vi "roboRIO TCP Client.vi"() -> ()   [LabVIEW 2025]
doc: "The UDP protocol differs from TCP in that there is no error-checking with the packets of information that are sent, and thus no guarantee whatsoever that an intended recipient will actually receive a given piece of data.\n\nUDP does offer the ability to \"broadcast\" data across a network--simply specify an IP Address of all ones (255.255.255.255) to attempt to broadcast information network-wide. Keep in mind that routers and other network hardware will generally refuse to forward the broadcast beyond certain points, so the extent of the broadcast will in practice be limited."
uses:
  roboRIO TCP Main States.ctl
panel:
  in  "Log?":bool
  out "Message Log":string[](array[string])
  out "String length":i32
  out "data string":string
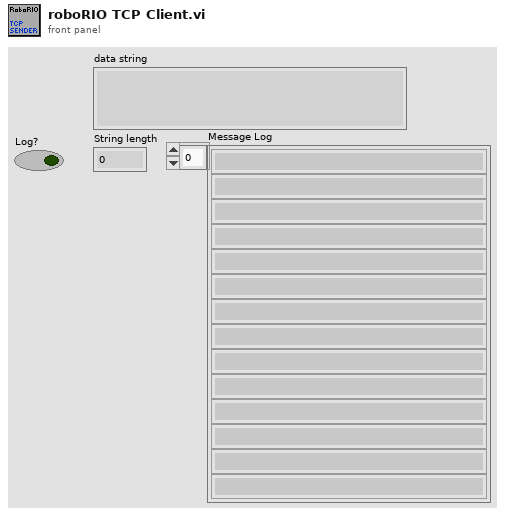
[diagram p1: front panel]
types:
  T1 = typedef "roboRIO TCP Main States.ctl" = enum16{"Message Dispatcher", "INI", "Read Data", "Send Data", "TCP Close", "TCP Open", "Exit"}
  T2 = typedef "Event Setup Types.ctl" = enum16{"Default", "Camera Loop Started", "GreyScale", "Reset Camera Settings", "Reset Team Number", "Save Data", "Setting Changed", "Update Video Mode", "Video Mode Changed", "Exit"}
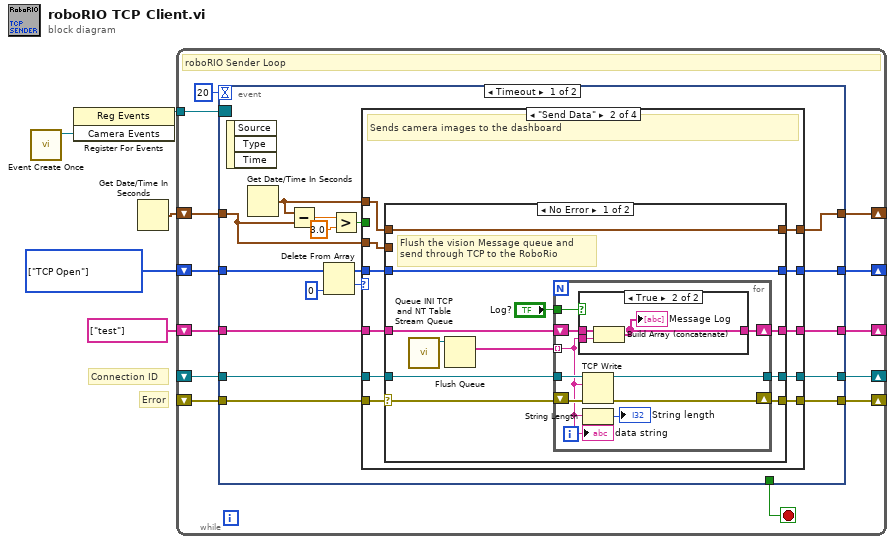
[diagram p0: block diagram]
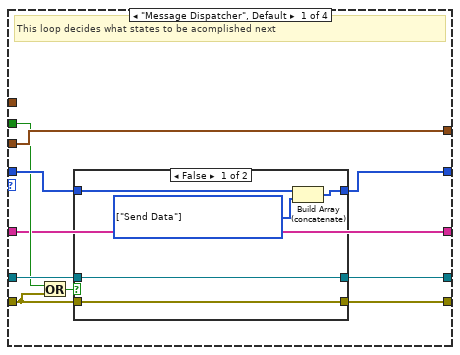
[diagram p2: hidden frame]
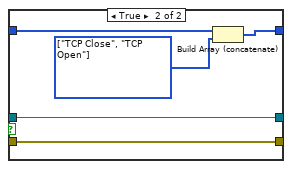
[diagram p3: hidden frame]
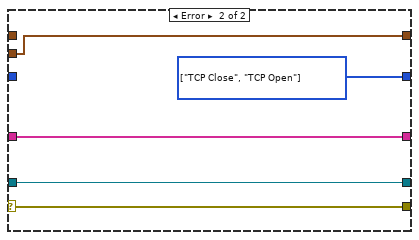
[diagram p5: hidden frame]
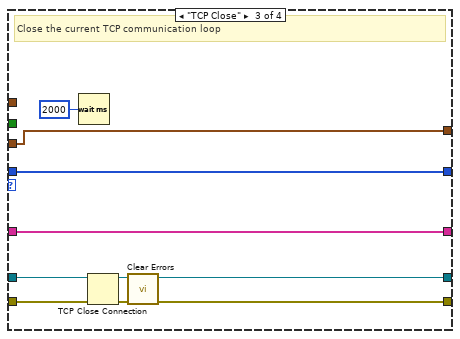
[diagram p6: hidden frame]
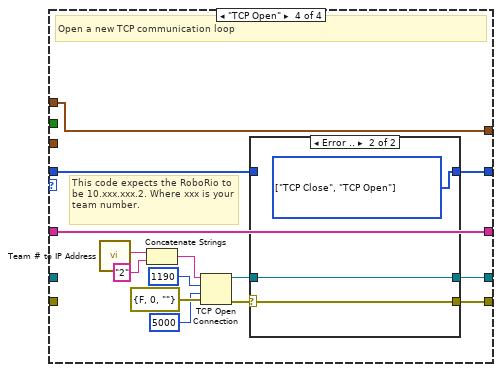
[diagram p7: hidden frame]
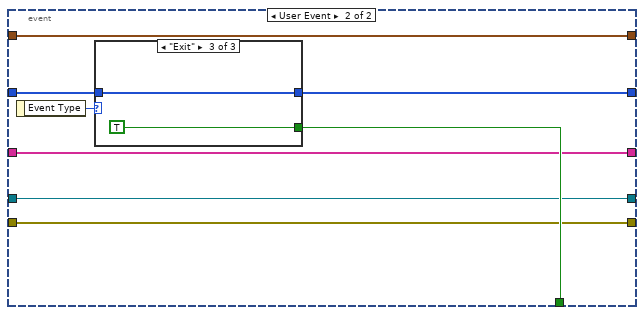
[diagram p9: hidden frame]
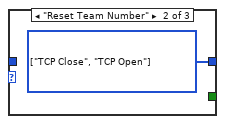
[diagram p11: hidden frame]
diagram:
  w5 = T1[] [enum."TCP Open"] items=["Message Dispatcher", "INI", "Read Data", "Send Data", "TCP Close", "TCP Open", "Exit"]
  # "Error"
  # "Connection ID"
  n1 = call "Event Create Once.vi"() -> ("Camera Events"=w3:refnum<user-event>)  [unwired: 10 in, 1 out]
  n2 = register-events(w3) -> (reference out=w2:refnum<event-registration>)  [unwired: 2 in, 1 out]
  n3 = Get Date/Time In Seconds() -> (seconds since 1Jan1904=w4:timestamp)
  n4 = while {
    shift-right: [w13] -> _
    shift-left: w5 -> [w14]
    shift-right: [w18] -> _
    shift-left: _ -> [w16]
    shift-right: [w17] -> _
    shift-left: _ -> [w15]
    shift-right: [w11] -> _
    shift-left: w4 -> [w10]
    tunnel: w2 -> [w9]
    shift-right: [w6] -> _
    shift-left: string[] ["test"] -> [w7]
    stop <- w12 stop-if-true
    # "roboRIO Sender Loop"
    n5 = event shown="[0] Timeout" {
      selector: w9 -> [_ _]
      dyn-events: _ -> [_ _]
      timeout: 20 -> [_ _]
      tunnel: [w35 w128] -> w18
      tunnel: [w34 w127] -> w17
      tunnel: w16 -> [w33 w128]
      tunnel: w15 -> [w20 w127]
      tunnel: w14 -> [w32 w129]
      tunnel: [w30 w126] -> w13
      tunnel: [_ w131] -> w12
      tunnel: [w24 w125] -> w11
      tunnel: w10 -> [w23 w125]
      tunnel: w7 -> [w22 w130]
      tunnel: [w21 w130] -> w6
      event Timeout {
        n6 = event-data() -> ()  [unwired: 1 in, 3 out]
        n7 = Get Date/Time In Seconds() -> (seconds since 1Jan1904=w25:timestamp)
        n8 = Subtract(x=w25, y=w23) -> (x-y=w28:dbl)
        n9 = Delete From Array(array=w32, index=0) -> (deleted portion=w19:T1, array with subset deleted=w31:T1[])  [unwired: 1 in]
        n10 = Greater?(x=w28, y=3.0) -> (0:w26:bool)
        n11 = case shown="\"Send Data\"" w19 {
          tunnel: [w42 w65 w99 w115] -> w35
          tunnel: [w40 w66 w100 w118] -> w34
          tunnel: w33 -> [w43 w64 w103 _]
          tunnel: w20 -> [w41 w61 w102 _]
          tunnel: w31 -> [w45 w63 w104 w117]
          tunnel: [w44 w62 w104 w116] -> w30
          tunnel: w26 -> [w38 _ _ _]
          tunnel: w25 -> [_ w60 _ w114]
          tunnel: [w39 w59 w97 w114] -> w24
          tunnel: w23 -> [w39 w58 w97 _]
          tunnel: w22 -> [w36 w57 w96 w109]
          tunnel: [w36 w56 w96 w109] -> w21
          frame "Message Dispatcher", Default {
            # "This loop decides what states to be acomplished next"
            n12 = Or(x=w38, y=w41) -> (x .or. y?=w37:bool)
            n13 = case shown="False" w37 {
              tunnel: [w46 w51] -> w40
              tunnel: w45 -> [w50 w55]
              tunnel: [w48 w53] -> w44
              tunnel: w43 -> [w49 w54]
              tunnel: [w49 w54] -> w42
              tunnel: w41 -> [w46 w51]
              frame False {
                w47 = T1[] [enum."Send Data"] items=["Message Dispatcher", "INI", "Read Data", "Send Data", "TCP Close", "TCP Open", "Exit"]
                n14 = Build Array (concatenate)(w50, w47) -> (w48:T1[])
              }
              frame True {
                w52 = T1[] [enum."TCP Close", enum."TCP Open"] items=["Message Dispatcher", "INI", "Read Data", "Send Data", "TCP Close", "TCP Open", "Exit"]
                n15 = Build Array (concatenate)(w55, w52) -> (w53:T1[])
              }
            }
          }
          frame "Send Data" {
            # "Sends camera images to the dashboard"
            n16 = case shown="No Error" w61 {
              selector: w61 -> [w73 w94]
              tunnel: [w77 w94] -> w66
              tunnel: [w76 w95] -> w65
              tunnel: w64 -> [w75 w95]
              tunnel: w63 -> [w74 _]
              tunnel: [w74 w93] -> w62
              tunnel: w60 -> [w72 _]
              tunnel: [w72 w92] -> w59
              tunnel: w58 -> [_ w92]
              tunnel: w57 -> [w71 w91]
              tunnel: [w70 w91] -> w56
              frame No Error {
                # "Flush the vision Message queue and send through TCP to the RoboRio"
                n17 = call "Queue INI TCP and NT Table Stream Queue.vi"() -> ("Queue out"=w69:refnum<queue>)  [unwired: 11 in]
                n18 = Flush Queue(queue=w69) -> (remaining elements=w68:string[])  [unwired: 1 in, 2 out]
                n19 = for {
                  tunnel: [w85] -> w76
                  tunnel: w75 -> [w84]
                  shift-right: [w86] -> w77
                  shift-left: w73 -> [w83]
                  tunnel: w68 -> [w79] mode=indexing
                  shift-right: [w80] -> w70
                  shift-left: w71 -> [w81]
                  tunnel: "Log?" -> [w78]
                  n20 = case shown="True" w78 {
                    tunnel: w81 -> [w87 w90]
                    tunnel: w79 -> [_ w89]
                    tunnel: [w87 w88] -> w80
                    frame False {
                    }
                    frame True {
                      n21 = Build Array (concatenate)(w90, w89) -> (w88:string[])
                      "Message Log" <- w88
                    }
                  }
                  n22 = TCP Write(connection ID=w84, data in=w79, error in (no error)=w83) -> (connection ID out=w85:refnum<k5>, error out=w86:errorcluster)  [unwired: 1 in, 1 out]
                  n23 = String Length(string=w79) -> (length=→"String length":i32)
                  "data string" <- w79
                }
              }
              frame Error {
                w93 = T1[] [enum."TCP Close", enum."TCP Open"] items=["Message Dispatcher", "INI", "Read Data", "Send Data", "TCP Close", "TCP Open", "Exit"]
              }
            }
          }
          frame "TCP Close" {
            # "Close the current TCP communication loop"
            n24 = Wait (ms)(milliseconds to wait=u32 2000) -> ()  [unwired: 1 out]
            n25 = TCP Close Connection(connection ID=w103, error in (no error)=w102) -> (connection ID out=w99:refnum<k5>, error out=w101:errorcluster)  [unwired: 1 in]
            n26 = call <vilib>:"Clear Errors.vi"("error in (no error)"=w101) -> ("error out"=w100:errorcluster)  [unwired: 5 in, 1 out]
          }
          frame "TCP Open" {
            # "This code expects the RoboRio to be 10.xxx.xxx.2. Where xxx is your team number."
            # "Open a new TCP communication loop"
            n27 = call "Team # to IP Address.vi"() -> ("Team IP Address"=w108:string)  [unwired: 11 in]
            n28 = Concatenate Strings(w108, "2" ("string")) -> (w106:string)
            n29 = TCP Open Connection(address=w106, remote port or service name=u16 1190 ("local port"), timeout ms (60000)=5000, error in (no error)=errorcluster {"status"=FALSE, "code"=0, "source"=""}) -> (connection ID=w111:refnum<k5>, error out=w112:errorcluster)  [unwired: 1 in]
            n30 = case shown="Error .." w112 {
              selector: w112 -> [w121 w123]
              tunnel: [w121 w123] -> w118
              tunnel: w117 -> [w120 _]
              tunnel: [w120 w124] -> w116
              tunnel: w111 -> [w119 w122]
              tunnel: [w119 w122] -> w115
              frame No Error {
              }
              frame Error {
                w124 = T1[] [enum."TCP Close", enum."TCP Open"] items=["Message Dispatcher", "INI", "Read Data", "Send Data", "TCP Close", "TCP Open", "Exit"]
              }
            }
          }
        }
      }
      event User Event {
        n31 = event-data() -> ("Event Type"=w132:T2)  [unwired: 1 in]
        n32 = case shown="\"Exit\"" w132 {
          tunnel: [_ _ TRUE] -> w131
          tunnel: w129 -> [w133 _ w135]
          tunnel: [w133 w134 w135] -> w126
          frame Default {
          }
          frame "Reset Team Number" {
            w134 = T1[] [enum."TCP Close", enum."TCP Open"] items=["Message Dispatcher", "INI", "Read Data", "Send Data", "TCP Close", "TCP Open", "Exit"]
          }
          frame "Exit" {
          }
        }
      }
    }
  }
